vi "读出所有测量记录.vi"() -> ()   [LabVIEW 2025]
panel:
  out "所有测量记录":string[][](table)
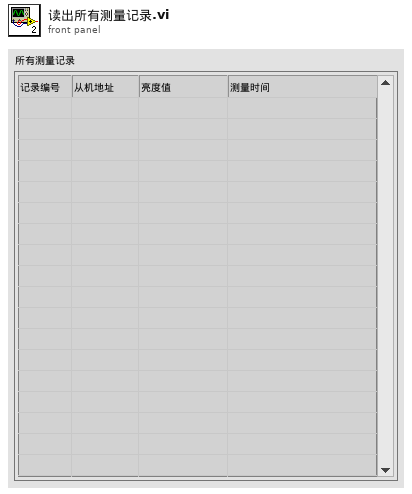
[diagram p1: front panel]
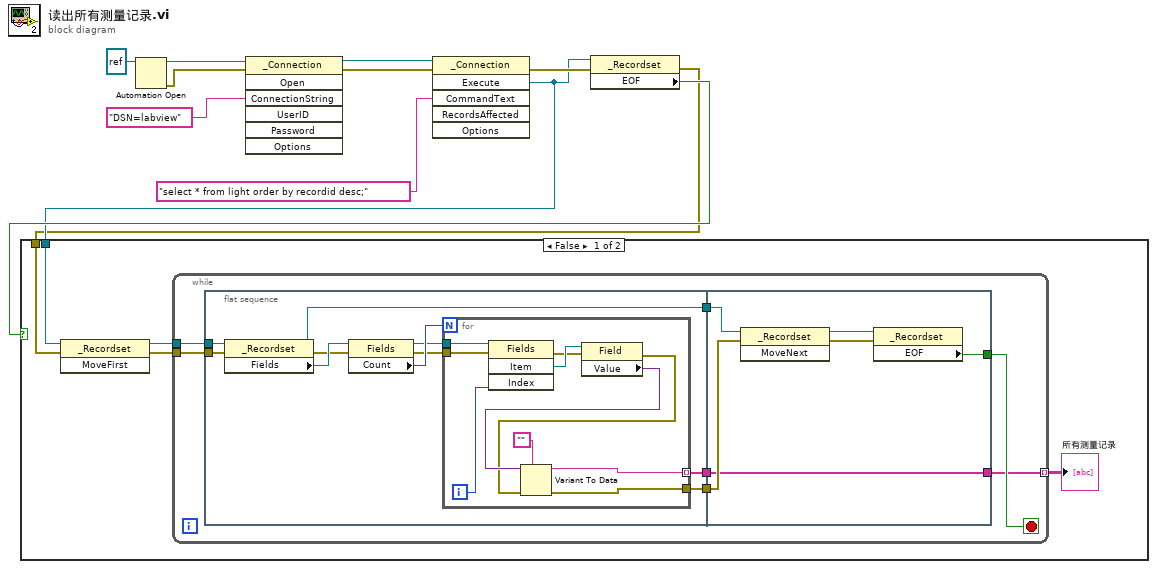
[diagram p0: block diagram]
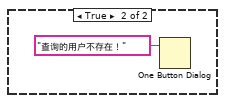
[diagram p2: hidden frame]
diagram:
  n1 = Automation Open(Automation Refnum=refnum<k7> refnum ("ADODB._Connection")) -> (Automation Refnum=w10:refnum<k7>, error out=w9:errorcluster)  [unwired: 3 in]
  n2 = invoke class="_Connection" method="Open"(reference=w10, error in=w9, "ConnectionString"="DSN=labview") -> (reference out=w7:refnum<k7>, error out=w6:errorcluster)  [unwired: 4 in, 5 out]
  n3 = invoke class="_Connection" method="Execute"(reference=w7, error in=w6, "CommandText"="select * from light order by recordid desc;") -> (error out=w4:errorcluster, "Execute"=w2:refnum<k7>)  [unwired: 3 in, 4 out]
  n4 = property class="_Recordset"(reference=w2, error in=w4) -> (error out=w1:errorcluster, "EOF"=w3:bool)  [unwired: 1 out]
  n5 = case shown="False" w3 {
    tunnel: w2 -> [w16 _]
    tunnel: w1 -> [w15 _]
    frame False {
      n6 = invoke class="_Recordset" method="MoveFirst"(reference=w16, error in=w15) -> (reference out=w13:refnum<k7>, error out=w14:errorcluster)  [unwired: 1 in, 1 out]
      n7 = while {
        tunnel: w14 -> [w21]
        tunnel: w13 -> [w20]
        tunnel: [w17] -> w12 mode=indexing
        stop <- w19 stop-if-true
        n8 = flat-sequence {
          tunnel: w20 -> [w33]
          tunnel: w21 -> [w32]
          tunnel: [w26] -> w23
          tunnel: [w25] -> w22
          tunnel: [w24] -> w18
          tunnel: w23 -> [w47]
          tunnel: w22 -> [w46]
          tunnel: [w45] -> w19
          tunnel: w18 -> [w44]
          tunnel: [w44] -> w17
          frame #0 {
            n9 = property class="_Recordset"(reference=w33, error in=w32) -> (reference out=w25:refnum<k7>, error out=w30:errorcluster, "Fields"=w31:refnum<k7>)
            n10 = property class="Fields"(reference=w31, error in=w30) -> (reference out=w28:refnum<k7>, error out=w27:errorcluster, "Count"=w29:i32)
            n11 = for {
              N: w29 -> [_]
              tunnel: w28 -> [w38]
              tunnel: w27 -> [w37]
              tunnel: [w35] -> w24 mode=indexing
              tunnel: [w34] -> w26
              i -> [w36]
              n12 = invoke class="Fields" method="Item"(reference=w38, error in=w37, "Index"=w36) -> (error out=w42:errorcluster, "Item"=w43:refnum<k7>)  [unwired: 1 in, 2 out]
              n13 = property class="Field"(reference=w43, error in=w42) -> (error out=w39:errorcluster, "Value"=w40:variant)  [unwired: 1 out]
              n14 = Variant To Data(error in=w39, type="", Variant=w40) -> (data=w35:string, error out=w34:errorcluster)
            }
          }
          frame #1 {
            n15 = invoke class="_Recordset" method="MoveNext"(reference=w46, error in=w47) -> (reference out=w49:refnum<k7>, error out=w48:errorcluster)  [unwired: 1 in, 1 out]
            n16 = property class="_Recordset"(reference=w49, error in=w48) -> ("EOF"=w45:bool)  [unwired: 2 out]
          }
        }
      }
      "所有测量记录" <- w12
    }
    frame True {
      n17 = One Button Dialog(message="查询的用户不存在！") -> ()  [unwired: 1 in, 1 out]
    }
  }
